vi "内置命令队列VI Tree.vi"   [LabVIEW 2012]
uses:
  <vilib>/CommandQueue/Command Queue.lvlib
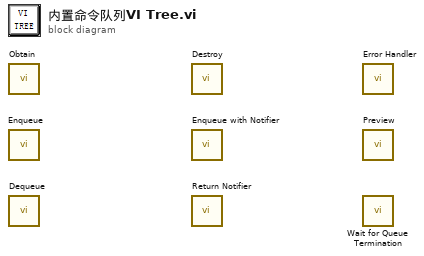
[diagram p0: block diagram]
diagram:
  n1 = call <vilib>:"Obtain.vi"() -> ()  [unwired: 9 in, 3 out]
  n2 = call <vilib>:"Enqueue.vi"() -> ()  [unwired: 9 in, 3 out]
  n3 = call <vilib>:"Dequeue.vi"() -> ()  [unwired: 7 in, 5 out]
  n4 = call <vilib>:"Destroy.vi"() -> ()  [unwired: 9 in, 3 out]
  n5 = call <vilib>:"Enqueue with Notifier.vi"() -> ()  [unwired: 9 in, 3 out]
  n6 = call <vilib>:"Return Notifier.vi"() -> ()  [unwired: 11 in, 1 out]
  n7 = call <vilib>:"Error Handler.vi"() -> ()  [unwired: 10 in, 2 out]
  n8 = call <vilib>:"Preview.vi"() -> ()  [unwired: 7 in, 5 out]
  n9 = call <vilib>:"Wait for Queue Termination.vi"() -> ()  [unwired: 11 in, 1 out]
